vi "parseCustomFlag1.vi"(8 "error in (no error)":errorcluster, 10 "Numeric":i8, 11 "Orion_BMS in":refnum<class "Orion_BMS.lvclass">) -> (0 "error out":errorcluster, 2 "output cluster":T1, 3 "Orion_BMS out":refnum<class "Orion_BMS.lvclass">)   [LabVIEW 2017, in "Orion_BMS.lvclass"]
uses:
  Orion_BMS.lvclass
  TypeDef_BMS_Status.ctl
  Orion_BMS.lvclass/Orion_BMS.ctl
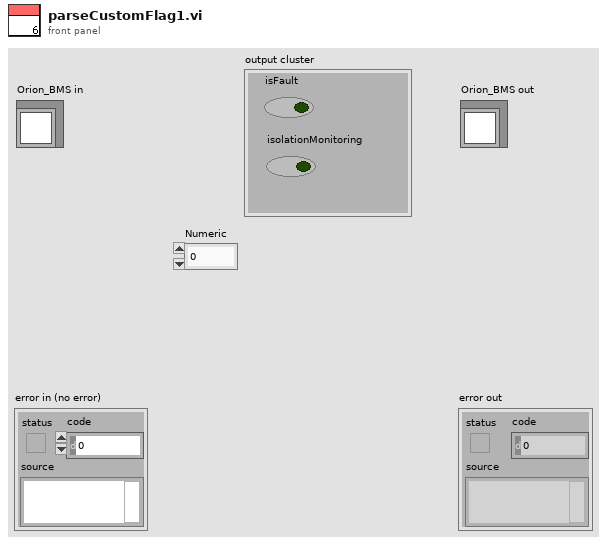
[diagram p1: front panel]
types:
  T1 = typedef "TypeDef_BMS_Status.ctl" = cluster{"isFault":bool, "isolationMonitoring":bool}
  T2 = typedef "TypeDef_BMSData.ctl" = cluster{"Max Cell Voltage (V)":dbl, "Max Cell ID":dbl, "Min Cell Voltage (V)":dbl, "Min Cell ID":dbl, "State of Charge (%)":dbl, "Average Voltage (V)":dbl, "Voltage Delta (V)":dbl, "Pack Current (A)":dbl, "Pack Voltage (V)":dbl, "Max Resistance (Ohm)":dbl, "Min Resistance (Ohm)":dbl, "Average Resistance (Ohm)":dbl, "Delta Resistance (Ohm)":dbl, "Highest Temperature(F)":dbl, "BmsStatus":T1}
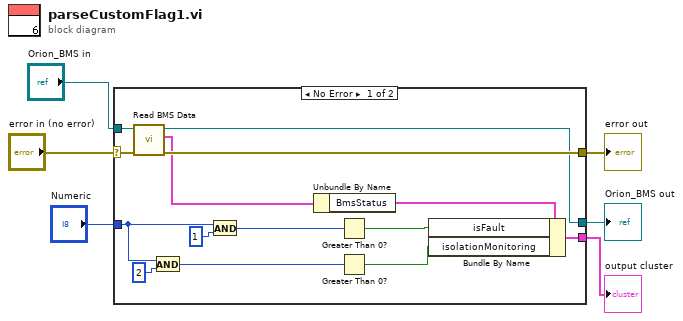
[diagram p0: block diagram]
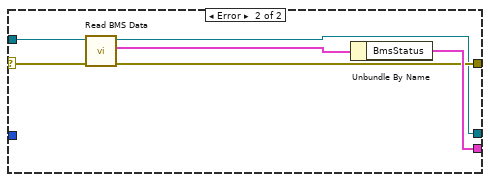
[diagram p2: hidden frame]
diagram:
  n1 = case shown="No Error" "error in (no error)" {
    selector: "error in (no error)" -> [w10 w24]
    tunnel: [w9 w22] -> w5
    tunnel: "Orion_BMS in" -> [w11 w25]
    tunnel: "Numeric" -> [w13 _]
    tunnel: [w16 w26] -> w2
    tunnel: [w7 w21] -> w1
    frame No Error {
      n2 = call "Read BMS Data.vi"("error in (no error)"=w10, "Orion_BMS in"=w11) -> ("error out"=w9:errorcluster, "BMS Data"=w8:T2, "Orion_BMS out"=w7:refnum<class "Orion_BMS.lvclass">)  [unwired: 7 in]
      n3 = And(x=w13, y=2) -> (x .and. y?=w15:i32)
      n4 = And(x=w13, y=1) -> (x .and. y?=w19:i32)
      n5 = Unbundle By Name(w8) -> ("BmsStatus"=w18:T1)
      n6 = Greater Than 0?(x=w19) -> (x > 0?=w17:bool)
      n7 = Greater Than 0?(x=w15) -> (x > 0?=w12:bool)
      n8 = Bundle By Name(cluster=w18, "isFault"=w17, "isolationMonitoring"=w12) -> (w16:T1)
    }
    frame Error {
      n9 = call "Read BMS Data.vi"("error in (no error)"=w24, "Orion_BMS in"=w25) -> ("error out"=w22:errorcluster, "BMS Data"=w23:T2, "Orion_BMS out"=w21:refnum<class "Orion_BMS.lvclass">)  [unwired: 7 in]
      n10 = Unbundle By Name(w23) -> ("BmsStatus"=w26:T1)
    }
  }
  "error out" <- w5
  "Orion_BMS out" <- w1
  "output cluster" <- w2
